vi "TestChromaPS.vi"() -> ()   [LabVIEW 2018]
panel:
  in  "Boolean":bool
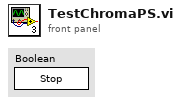
[diagram p1: front panel]
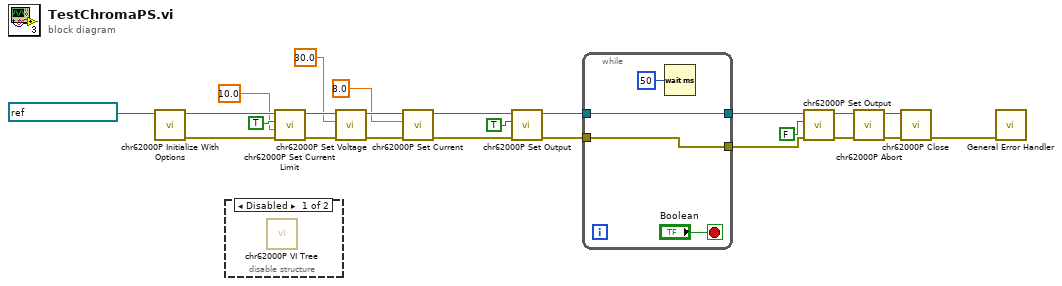
[diagram p0: block diagram]
diagram:
  n1 = call <instrlib>:"chr62000P Initialize With Options.vi"("resource name"=refnum<k15> "CHROMAOUT0") -> ("error out"=w15:errorcluster, "instrument handle out"=w16:refnum<k15>)  [unwired: 9 in]
  n2 = disable-structure shown="Disabled" {
    frame Disabled {
      n3 = call <instrlib>:"chr62000P VI Tree.vi"() -> ()  [unwired: 12 in]
    }
    frame Enabled {
    }
  }
  n4 = call <instrlib>:"chr62000P Set Current Limit.vi"("error in (no error)"=w15, "Current Limit (0.0)"=10.0, "High/Low (Low)"=TRUE, "instrument handle"=w16) -> ("error out"=w14:errorcluster, "instrument handle out"=w24:refnum<k15>)  [unwired: 6 in]
  n5 = call <instrlib>:"chr62000P Set Voltage.vi"("error in (no error)"=w14, "Voltage (0.00)"=30.0, "instrument handle"=w24) -> ("error out"=w4:errorcluster, "instrument handle out"=w6:refnum<k15>)  [unwired: 7 in]
  n6 = call <instrlib>:"chr62000P Set Current.vi"("error in (no error)"=w4, "Current (0.00)"=8.0, "instrument handle"=w6) -> ("error out"=w3:errorcluster, "instrument handle out"=w5:refnum<k15>)  [unwired: 7 in]
  n7 = call <instrlib>:"chr62000P Set Output.vi"("error in (no error)"=w3, "Output (Off)"=TRUE, "instrument handle"=w5) -> ("error out"=w8:errorcluster, "instrument handle out"=w11:refnum<k15>)  [unwired: 7 in]
  n8 = while {
    tunnel: w11 -> [w28]
    tunnel: [w28] -> w10
    tunnel: [w27] -> w9
    tunnel: w8 -> [w27]
    stop <- "Boolean" stop-if-true
    n9 = Wait (ms)(milliseconds to wait=u32 50) -> ()  [unwired: 1 out]
  }
  n10 = call <instrlib>:"chr62000P Set Output.vi"("error in (no error)"=w9, "Output (Off)"=FALSE, "instrument handle"=w10) -> ("error out"=w19:errorcluster, "instrument handle out"=w20:refnum<k15>)  [unwired: 7 in]
  n11 = call <instrlib>:"chr62000P Abort.vi"("error in (no error)"=w19, "instrument handle"=w20) -> ("error out"=w17:errorcluster, "instrument handle out"=w18:refnum<k15>)  [unwired: 8 in]
  n12 = call <instrlib>:"chr62000P Close.vi"("error in (no error)"=w17, "instrument handle"=w18) -> ("error out"=w13:errorcluster)  [unwired: 9 in]
  n13 = call <vilib>:"General Error Handler.vi"("error in (no error)"=w13) -> ()  [unwired: 10 in, 5 out]
